vi "Revision Query.vi"(8 "error in (no error)":errorcluster {"code" format="%.0x"}, 9 "Buffer size (256)":i32=256, 11 "instrument handle":refnum<k15>) -> (0 "error out":errorcluster {"code" format="%.0x"}, 1 "firmware revision":string, 2 "instrument driver revision":string, 3 "instrument handle out":refnum<k15>)   [LabVIEW 2009, in "Keysight XSAn.lvlib"]
doc: "Retrieves revision information from the instrument."
uses:
  <instrlib>/Keysight XSAn/Keysight XSAn.lvlib
  AgXSAn.dll
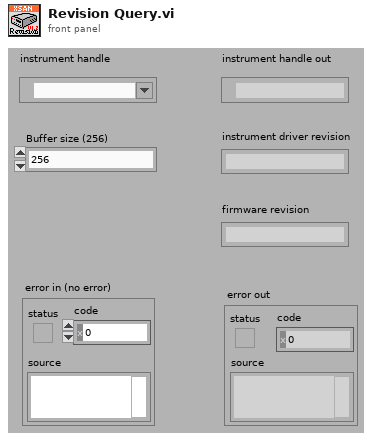
[diagram p1: front panel]
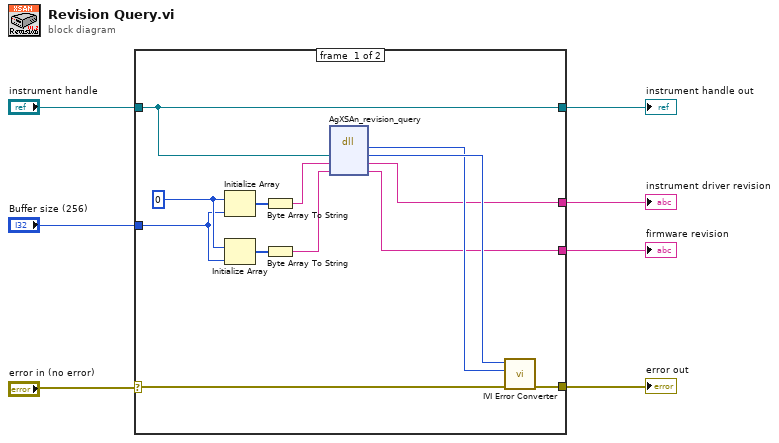
[diagram p0: block diagram]
diagram:
  n1 = case shown="No Error" "error in (no error)" {
    selector: "error in (no error)" -> [w14 w22]
    tunnel: [w15 w22] -> w6
    tunnel: "instrument handle" -> [w9 w21]
    tunnel: [w11 _] -> w4
    tunnel: [w10 _] -> w3
    tunnel: [w9 w21] -> w2
    tunnel: "Buffer size (256)" -> [w8 _]
    frame #0 {
      w12 = u8 0
      n2 = Initialize Array(w12, w8) -> (w20:u8[])
      n3 = Initialize Array(w12, w8) -> (w19:u8[])
      n4 = Byte Array To String(unsigned byte array=w20) -> (string=w18:string)
      n5 = Byte Array To String(unsigned byte array=w19) -> (string=w17:string)
      n6 = dll-call lib="AgXSAn**.dll" fn="AgXSAn_revision_query" ("LabVIEW:IviSpecAn_revision_query")("instrument handle"=w9, "instrument driver revision"=w18, "firmware revision"=w17) -> ("Status"=w13:i32, "instrument handle"=w16:u32, "instrument driver revision"=w10:string, "firmware revision"=w11:string)  [unwired: 3 in, 2 out]
      n7 = call <instrlib>:"IVI Error Converter.vi"("error in (no error)"=w14, "IVI error code (0)"=w13, "instrument handle"=w16) -> ("error out"=w15:errorcluster)  [unwired: 7 in, 1 out]
    }
    frame #1 {
    }
  }
  "error out" <- w6
  "instrument handle out" <- w2
  "firmware revision" <- w4
  "instrument driver revision" <- w3
